vi "DAQ.PreStartWriteBuffer.vi"(8 "error in (no error)":errorcluster, 11 "Instrument.DAQ in":refnum<class "Instrument.DAQ.lvclass">) -> (0 "error out":errorcluster, 3 "Instrument.DAQ out":refnum<class "Instrument.DAQ.lvclass">)   [LabVIEW 2019, in "Instrument.Lockin.lvlib" / "Instrument.DAQ.lvclass"]
uses:
  Instrument.DAQ.lvclass
  Typedefs/Sweep.State--enum.ctl
  Instrument.DAQ.lvclass/Instrument.DAQ.ctl
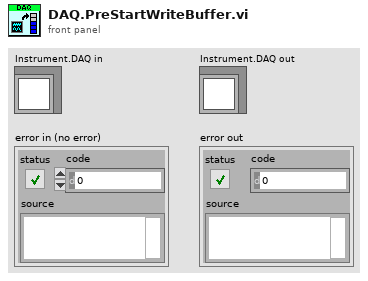
[diagram p1: front panel]
types:
  T1 = typedef "Instrument.Lockin.lvlib/Instrument.DAQ.lvclass/Sweep.State--enum.ctl" = enum16{"idle", "initialize", "wait", "sweep", "stop"}
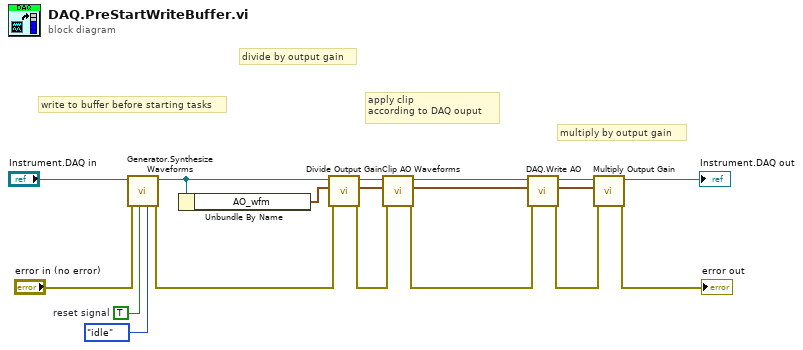
[diagram p0: block diagram]
diagram:
  w3 = TRUE  # reset signal
  # "multiply by output gain"
  # "write to buffer before starting tasks"
  # "apply clip\naccording to DAQ ouput"
  # "divide by output gain"
  n1 = call "Generator.Synthesize Waveforms.vi"("sweep state"=Sweep.State--enum."idle", "Reset Phase?"=w3, "error in (no error)"="error in (no error)", "Instrument.DAQ"="Instrument.DAQ in") -> ("error out"=w7:errorcluster, "Instrument.DAQ"=w8:refnum<class "Instrument.DAQ.lvclass">)  [unwired: 6 in]
  n2 = Unbundle By Name(w8) -> ("AO_wfm"=w9:waveform(dbl)[])
  n3 = call "Divide Output Gain.vi"("error in (no error)"=w7, "WFM in"=w9, "Instrument.DAQ"=w8) -> ("error out"=w6:errorcluster, "WFM out"=w4:waveform(dbl)[], "Instrument.DAQ out"=w5:refnum<class "Instrument.DAQ.lvclass">)  [unwired: 6 in]
  n4 = call "Clip AO Waveforms.vi"("error in (no error)"=w6, "AO []"=w4, "Instrument.DAQ in"=w5) -> ("error out"=w17:errorcluster, "Clipped AO []"=w16:waveform(dbl)[], "Instrument.DAQ out"=w15:refnum<class "Instrument.DAQ.lvclass">)  [unwired: 6 in]
  n5 = call "DAQ.Write AO.vi"("error in (no error)"=w17, "AO []"=w16, "Instrument.DAQ in"=w15) -> ("error out"=w13:errorcluster, "AO out []"=w12:waveform(dbl)[], "Instrument.DAQ out"=w11:refnum<class "Instrument.DAQ.lvclass">)  [unwired: 5 in, 1 out]
  n6 = call "Multiply Output Gain.vi"("error in (no error)"=w13, "WFM in"=w12, "Instrument.DAQ"=w11) -> ("error out"=→"error out":errorcluster, "Instrument.DAQ out"=→"Instrument.DAQ out":refnum<class "Instrument.DAQ.lvclass">)  [unwired: 6 in, 1 out]
